vi "Create Topic Rule.vi"(8 "error in (no error)":errorcluster, 9 "Topic Rule":T1, 10 "Rule Name":string, 11 "IoT Session in":refnum<class "IoT Session.lvclass">) -> (0 "error out":errorcluster, 3 "IoT Session out":refnum<class "IoT Session.lvclass">)   [LabVIEW 2015, in "NI_AWS_IoT.lvlib" / "IoT Session.lvclass"]
uses:
  IoT Session.lvclass
  Topic Rule.ctl
  CloudWatch Alarm.ctl
  CloudWatch Metric.ctl
  DynamoDB.ctl
  DynamoDBv2.ctl
  Elasticsearch.ctl
  Firehose.ctl
  Kinesis.ctl
  Lambda.ctl
  Republish.ctl
  S3.ctl
  SNS.ctl
  SQS.ctl
  Core/HTTP Request/Valid String Specification.ctl
  Core/HTTP Request/Request Options.ctl
  Core/HTTP Request/Name Value Pair.ctl
  Core/HTTP Request/Region handling.ctl
  Core/HTTP Request/URL formatting.ctl
  Core/HTTP Request/HTTP Request.lvclass
  NI_AWS_IoT.lvlib
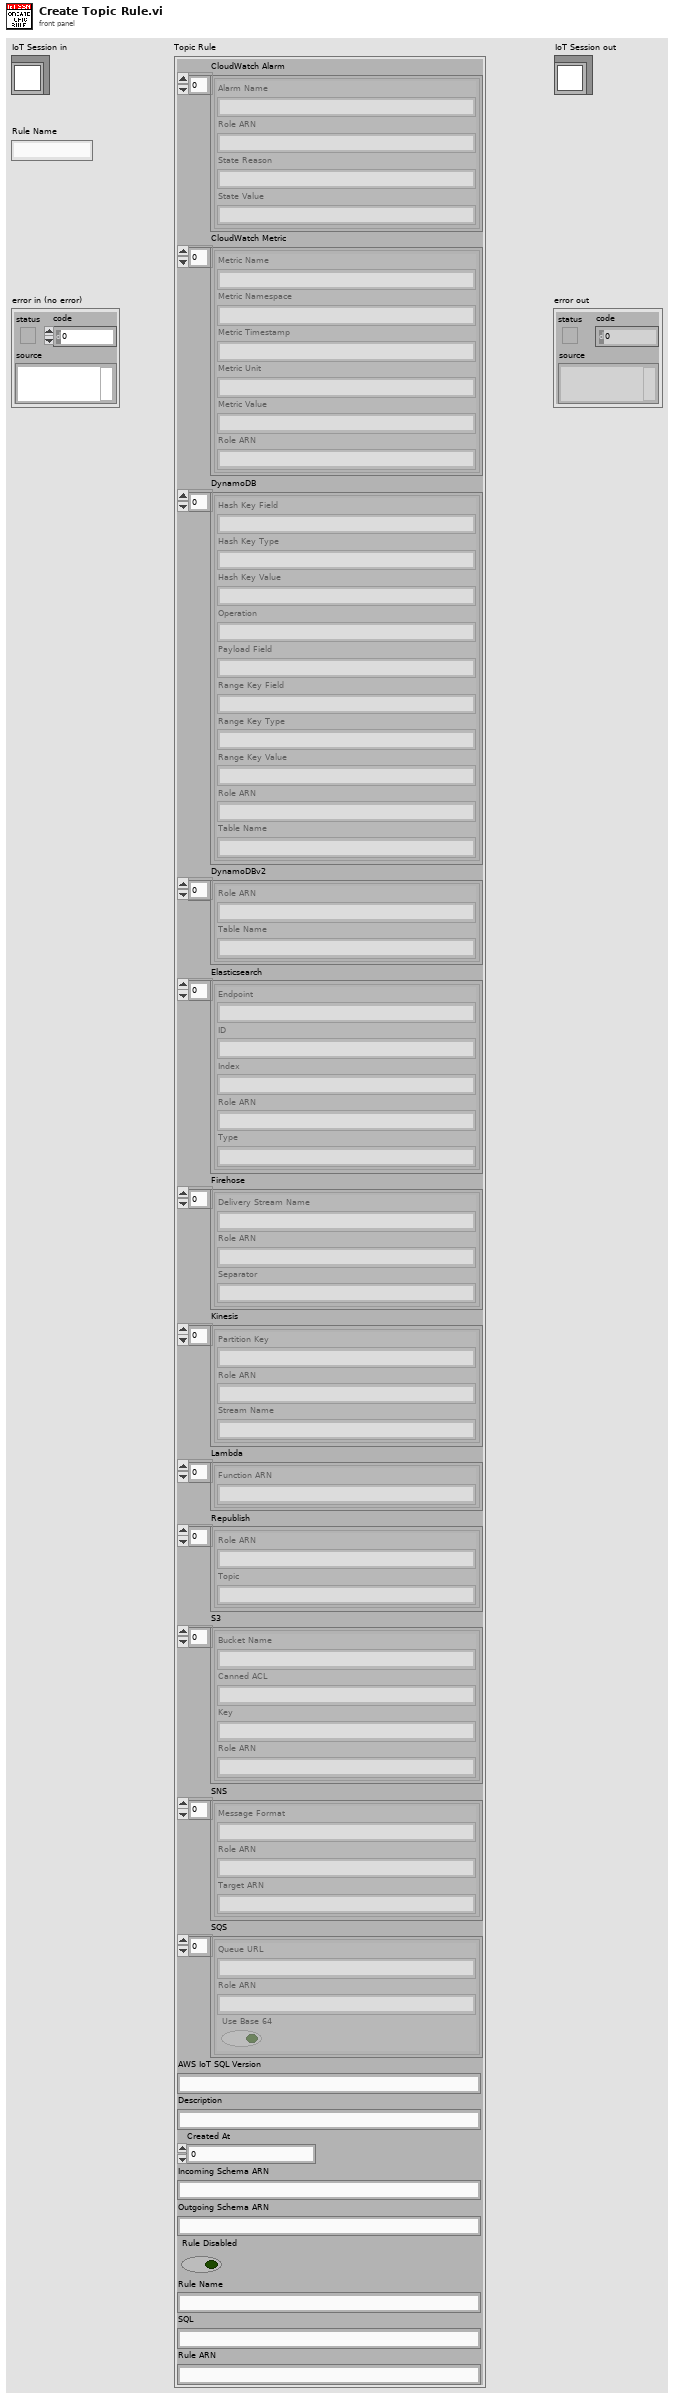
[diagram p1: front panel]
types:
  T1 = typedef "NI_AWS_IoT.lvlib/Topic Rule.ctl" = cluster{"CloudWatch Alarm":T2[], "CloudWatch Metric":T3[], "DynamoDB":T4[], "DynamoDBv2":T5[], "Elasticsearch":T6[], "Firehose":T7[], "Kinesis":T8[], "Lambda":T9[], "Republish":T10[], "S3":T11[], "SNS":T12[], "SQS":T13[], "AWS IoT SQL Version":string, "Description":string, "Created At":u64, "Incoming Schema ARN":string, "Outgoing Schema ARN":string, "Rule Disabled":bool, "Rule Name":string, "SQL":string, "Rule ARN":string}
  T2 = typedef "NI_AWS_IoT.lvlib/CloudWatch Alarm.ctl" = cluster{"Alarm Name":string, "Role ARN":string, "State Reason":string, "State Value":string}
  T3 = typedef "NI_AWS_IoT.lvlib/CloudWatch Metric.ctl" = cluster{"Metric Name":string, "Metric Namespace":string, "Metric Timestamp":string, "Metric Unit":string, "Metric Value":string, "Role ARN":string}
  T4 = typedef "NI_AWS_IoT.lvlib/DynamoDB.ctl" = cluster{"Hash Key Field":string, "Hash Key Type":string, "Hash Key Value":string, "Operation":string, "Payload Field":string, "Range Key Field":string, "Range Key Type":string, "Range Key Value":string, "Role ARN":string, "Table Name":string}
  T5 = typedef "NI_AWS_IoT.lvlib/DynamoDBv2.ctl" = cluster{"Role ARN":string, "Table Name":string}
  T6 = typedef "NI_AWS_IoT.lvlib/Elasticsearch.ctl" = cluster{"Endpoint":string, "ID":string, "Index":string, "Role ARN":string, "Type":string}
  T7 = typedef "NI_AWS_IoT.lvlib/Firehose.ctl" = cluster{"Delivery Stream Name":string, "Role ARN":string, "Separator":string}
  T8 = typedef "NI_AWS_IoT.lvlib/Kinesis.ctl" = cluster{"Partition Key":string, "Role ARN":string, "Stream Name":string}
  T9 = typedef "NI_AWS_IoT.lvlib/Lambda.ctl" = cluster{"Function ARN":string}
  T10 = typedef "NI_AWS_IoT.lvlib/Republish.ctl" = cluster{"Role ARN":string, "Topic":string}
  T11 = typedef "NI_AWS_IoT.lvlib/S3.ctl" = cluster{"Bucket Name":string, "Canned ACL":string, "Key":string, "Role ARN":string}
  T12 = typedef "NI_AWS_IoT.lvlib/SNS.ctl" = cluster{"Message Format":string, "Role ARN":string, "Target ARN":string}
  T13 = typedef "NI_AWS_IoT.lvlib/SQS.ctl" = cluster{"Queue URL":string, "Role ARN":string, "Use Base 64":bool}
  T14 = typedef "NI_AWS_Core.lvlib/HTTP Request.lvclass/Valid String Specification.ctl" = enum16{"none", "only [alphanumeric][-][_]", "only [alphanumeric][-][_][space]", "phone number +1xxxyyyzzzz", "Regular Expression"}
  T15 = typedef "NI_AWS_Core.lvlib/HTTP Request.lvclass/Name Value Pair.ctl" = cluster{"name":string, "value":string}
  T16 = typedef "NI_AWS_Core.lvlib/HTTP Request.lvclass/Request Options.ctl" = cluster{"request headers":T15[], "request parameters":T15[], "request body":string, "region handling":T17, "URL formatting":T18}
  T17 = typedef "NI_AWS_Core.lvlib/HTTP Request.lvclass/Region handling.ctl" = enum16{"use region everywhere", "use region (authentication only)", "use region (URL only)", "ignore region everwhere"}
  T18 = typedef "NI_AWS_Core.lvlib/HTTP Request.lvclass/URL formatting.ctl" = enum16{"region-", "region."}
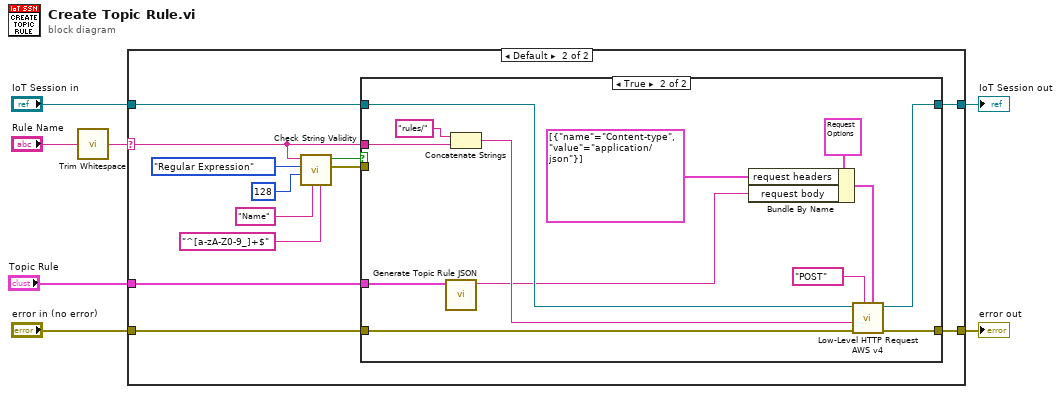
[diagram p0: block diagram]
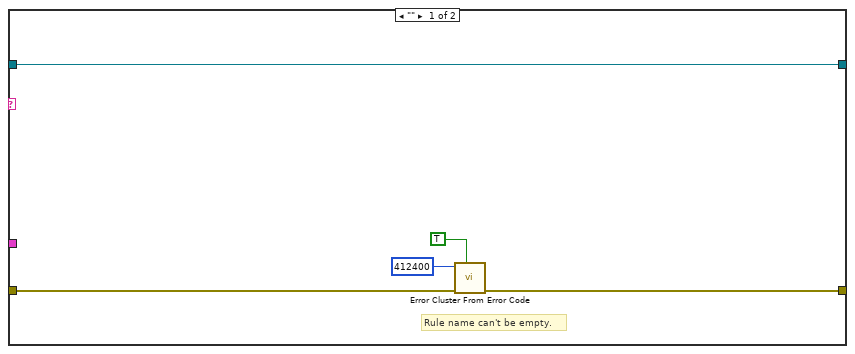
[diagram p2: hidden frame]
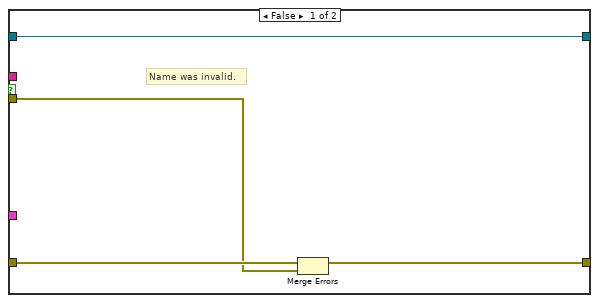
[diagram p3: hidden frame]
diagram:
  n1 = call <vilib>:"Trim Whitespace.vi"("string"="Rule Name") -> ("trimmed string"=w1:string)  [unwired: 1 in]
  n2 = case shown="Default" w1 {
    selector: w1 -> [_ w13]
    tunnel: "error in (no error)" -> [w9 w24]
    tunnel: [w8 w23] -> w6
    tunnel: [w12 w22] -> w5
    tunnel: "IoT Session in" -> [w12 w21]
    tunnel: "Topic Rule" -> [_ w20]
    frame "" {
      # "Rule name can't be empty."
      n3 = call <vilib>:"Error Cluster From Error Code.vi"("show call chain? (False)"=TRUE, "error in (no error)"=w9, "error code (0)"=412400) -> ("error out"=w8:errorcluster)  [unwired: 6 in]
    }
    frame Default {
      n4 = call "Check String Validity.vi"("Regular Expression"="^[a-zA-Z0-9_]+$", "String Name for Error"="Name", "Max Characters"=128, "Valid String Specification"=Valid_String_Specification."Regular Expression", "String"=w13) -> ("string error"=w14:errorcluster, "Valid"=w15:bool)  [unwired: 5 in]
      n5 = case shown="True" w15 {
        tunnel: w24 -> [w28 w39]
        tunnel: [w27 w38] -> w23
        tunnel: [w25 w37] -> w22
        tunnel: w21 -> [w25 w36]
        tunnel: w13 -> [_ w35]
        tunnel: w20 -> [_ w32]
        tunnel: w14 -> [w26 _]
        frame False {
          # "Name was invalid."
          n6 = Merge Errors(w28, w26) -> (w27:errorcluster)
        }
        frame True {
          n7 = call "Generate Topic Rule JSON.vi"("Topic Rule"=w32) -> ("Topic Rule JSON"=w29:string)  [unwired: 10 in]
          n8 = Concatenate Strings("rules/" ("string"), w35) -> (w33:string)
          n9 = Bundle By Name(cluster=T16 {"request headers"=[], "request parameters"=[], "request body"="", "region handling"=enum."use region everywhere", "URL formatting"=enum."region."} ("Request Options"), "request headers"=T15[] [{"name"="Content-type", "value"="application/json"}], "request body"=w29) -> (w40:T16)
          n10 = call "Low-Level HTTP Request AWS v4.vi"("Request Options"=w40, "HTTP-Verb"="POST", "error in (no error)"=w39, "URL Suffix"=w33, "AWS Core in"=w36) -> ("error out"=w38:errorcluster, "AWS Core out"=w37:refnum<class "IoT Session.lvclass">)  [unwired: 3 in, 2 out]
        }
      }
    }
  }
  "error out" <- w6
  "IoT Session out" <- w5
